vi "string2string_frame(SubVI).vi"(11 "String in":string) -> (3 "String out":string)   [LabVIEW 2012]
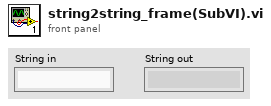
[diagram p1: front panel]
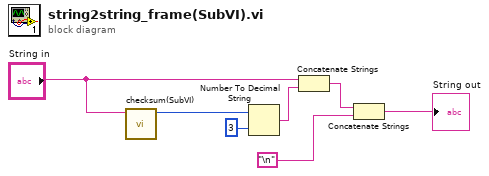
[diagram p0: block diagram]
diagram:
  n1 = call "checksum(SubVI).vi"("String"="String in") -> ("Numeric"=w2:u8)  [unwired: 10 in]
  n2 = Number To Decimal String(number=w2, width (-)=3) -> (decimal integer string=w4:string)
  n3 = Concatenate Strings("String in", w4) -> (w5:string)
  n4 = Concatenate Strings(w5, "\n") -> (→"String out":string)
